vi "Project_Final_2016.vi"() -> ()   [LabVIEW 2015]
uses:
  <vilib>/DAQmx/read.llb/DAQmx Read (Digital Bool 1Line 1Point).vi
  <vilib>/DAQmx/write.llb/DAQmx Write (Digital Bool 1Line 1Point).vi
  <vilib>/DAQmx/create/channels.llb/DAQmx Create Channel (DI-Digital Input).vi
  <vilib>/DAQmx/create/channels.llb/DAQmx Create Channel (DO-Digital Output).vi
  <vilib>/DAQmx/miscellaneous.llb/DAQmx Fill In Error Info.vi
  <vilib>/Utility/file.llb/Read Delimited Spreadsheet (DBL).vi
  <vilib>/Utility/file.llb/Write Delimited Spreadsheet (DBL).vi
panel:
  out "Reject area solenoid return":bool=TRUE
  out "Rejecting \nBelt Solenoid":bool
  out "Rotary Solenoid":bool
  out "Solenoid Return Sensor":bool=TRUE
  out "Sorting \nChain Solenoid":bool
  in  "BELT":bool
  in  "CHAIN":bool
  in  "PAUSE":bool
  in  "On/Off":bool
  out "cluster 2":T1
  out "ARRAY 2":dbl[](array[numeric])
  in  "Destination 2":path=path "C:/Users/dnt4/Downloads/data2.txt"
  out "ARRAY":dbl[](array[numeric])
  out "output cluster 2":T2
  out "output cluster":T3
  out "cluster":T4
  out "sensing area peg detect fake":bool
  in  "stop 4":bool
  in  "Assist sensing loop1 3":bool
  out "reject wait":dbl
  out "reject assistant":dbl
  in  "Assist sensing loop1 2":bool
  out "protection":dbl
  in  "stop 3":bool
  out "Assembly detect fake":bool
  out "Emergency Stop ACTIVATED":bool
  in  "Store Values":bool
  in  "Restore Values":bool
  out "Fake Emergency stop":bool
  out "% Efficiency":dbl(slide) scale=0.0..1.0 scale format="%.2f"
  in  "Clear":bool
  in  "stop 2":bool
  in  "Power Failure":bool
  out "array 2":dbl[](array[numeric])
  in  "Destination 1":path=path "C:/Users/dnt4/Downloads/data1.txt"
  out "array":dbl[](array[numeric])
  out "Stopped":bool=TRUE
  in  "stop AddOn Reject 1":bool
  out "Assembly Assist":dbl
  in  "Assist sensing loop1":bool
  in  "stop sensing station":bool
  out "Assembly Detect":bool
  out "# of Assembly Made":dbl(slide) scale=0.0..20.0
  out "# of Rings Rejected":dbl(slide) scale=0.0..20.0
  out "# of Peg Rejected":dbl(slide) scale=0.0..20.0
  out "# of Ring in the chute":dbl(slide) scale=0.0..5.0
  in  "stop reject area":bool
  out "Reject Area Detected":bool
  out "Sensing Area\n Peg Detected":bool
  out "Sensing Area \nRing Detected":bool
  in  "stop sensing area":bool
  out "Hopper is FULL":bool=TRUE
  in  "stop assembly chute":bool
  out "Sorting Area \nPeg detect":bool
  out "Sorting Area \nPart Detect":bool
  out "Running":bool
  in  "stop":bool
  # "Industrial Control  Trainer (ICT) USER CONTROL PANEL"
  # "Solenoid Activity"
  # "DATA STORAGE LOCATION"
  # "CHAIN/BELT CONTROL"
  # "Main Control"
  # "Sensor Activities"
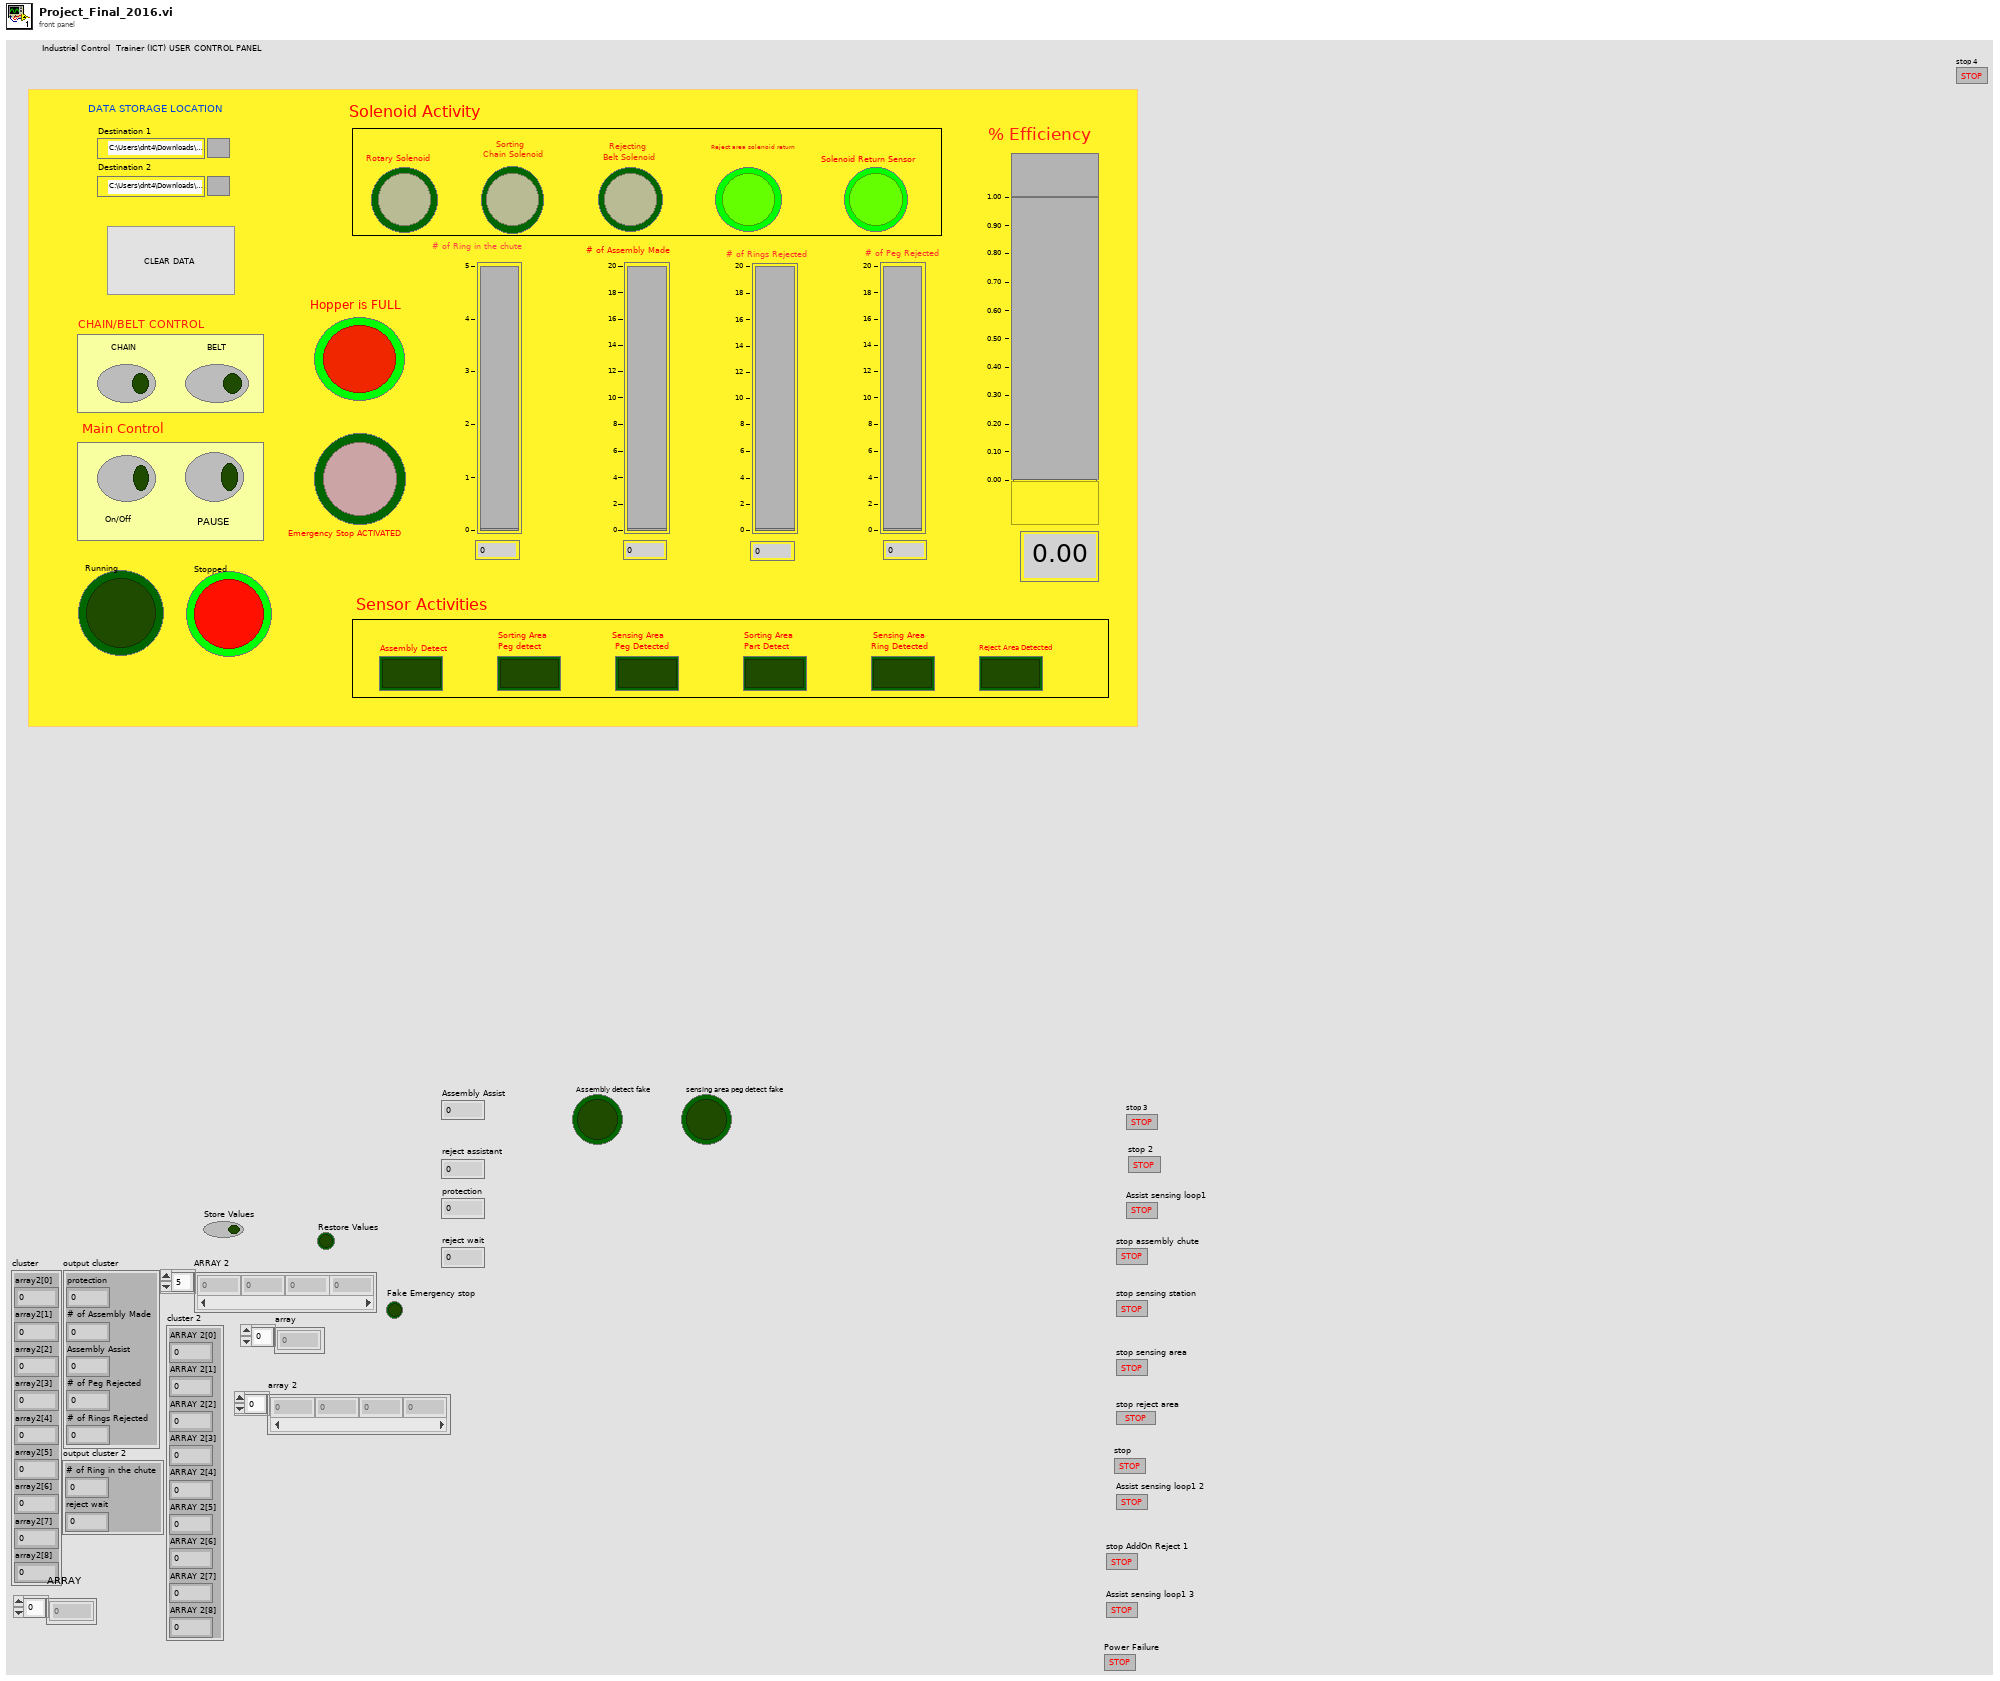
[diagram p1: front panel]
types:
  T1 = cluster{"ARRAY 2[0]":dbl, "ARRAY 2[1]":dbl, "ARRAY 2[2]":dbl, "ARRAY 2[3]":dbl, "ARRAY 2[4]":dbl, "ARRAY 2[5]":dbl, "ARRAY 2[6]":dbl, "ARRAY 2[7]":dbl, "ARRAY 2[8]":dbl}
  T2 = cluster{"# of Ring in the chute":dbl, "reject wait":dbl}
  T3 = cluster{"protection":dbl, "# of Assembly Made":dbl, "Assembly Assist":dbl, "# of Peg Rejected":dbl, "# of Rings Rejected":dbl}
  T4 = cluster{"array2[0]":dbl, "array2[1]":dbl, "array2[2]":dbl, "array2[3]":dbl, "array2[4]":dbl, "array2[5]":dbl, "array2[6]":dbl, "array2[7]":dbl, "array2[8]":dbl}
  T5 = cluster{"array 2[0]":dbl, "array 2[1]":dbl, "array 2[2]":dbl, "array 2[3]":dbl, "array 2[4]":dbl, "array 2[5]":dbl, "array 2[6]":dbl, "array 2[7]":dbl, "array 2[8]":dbl}
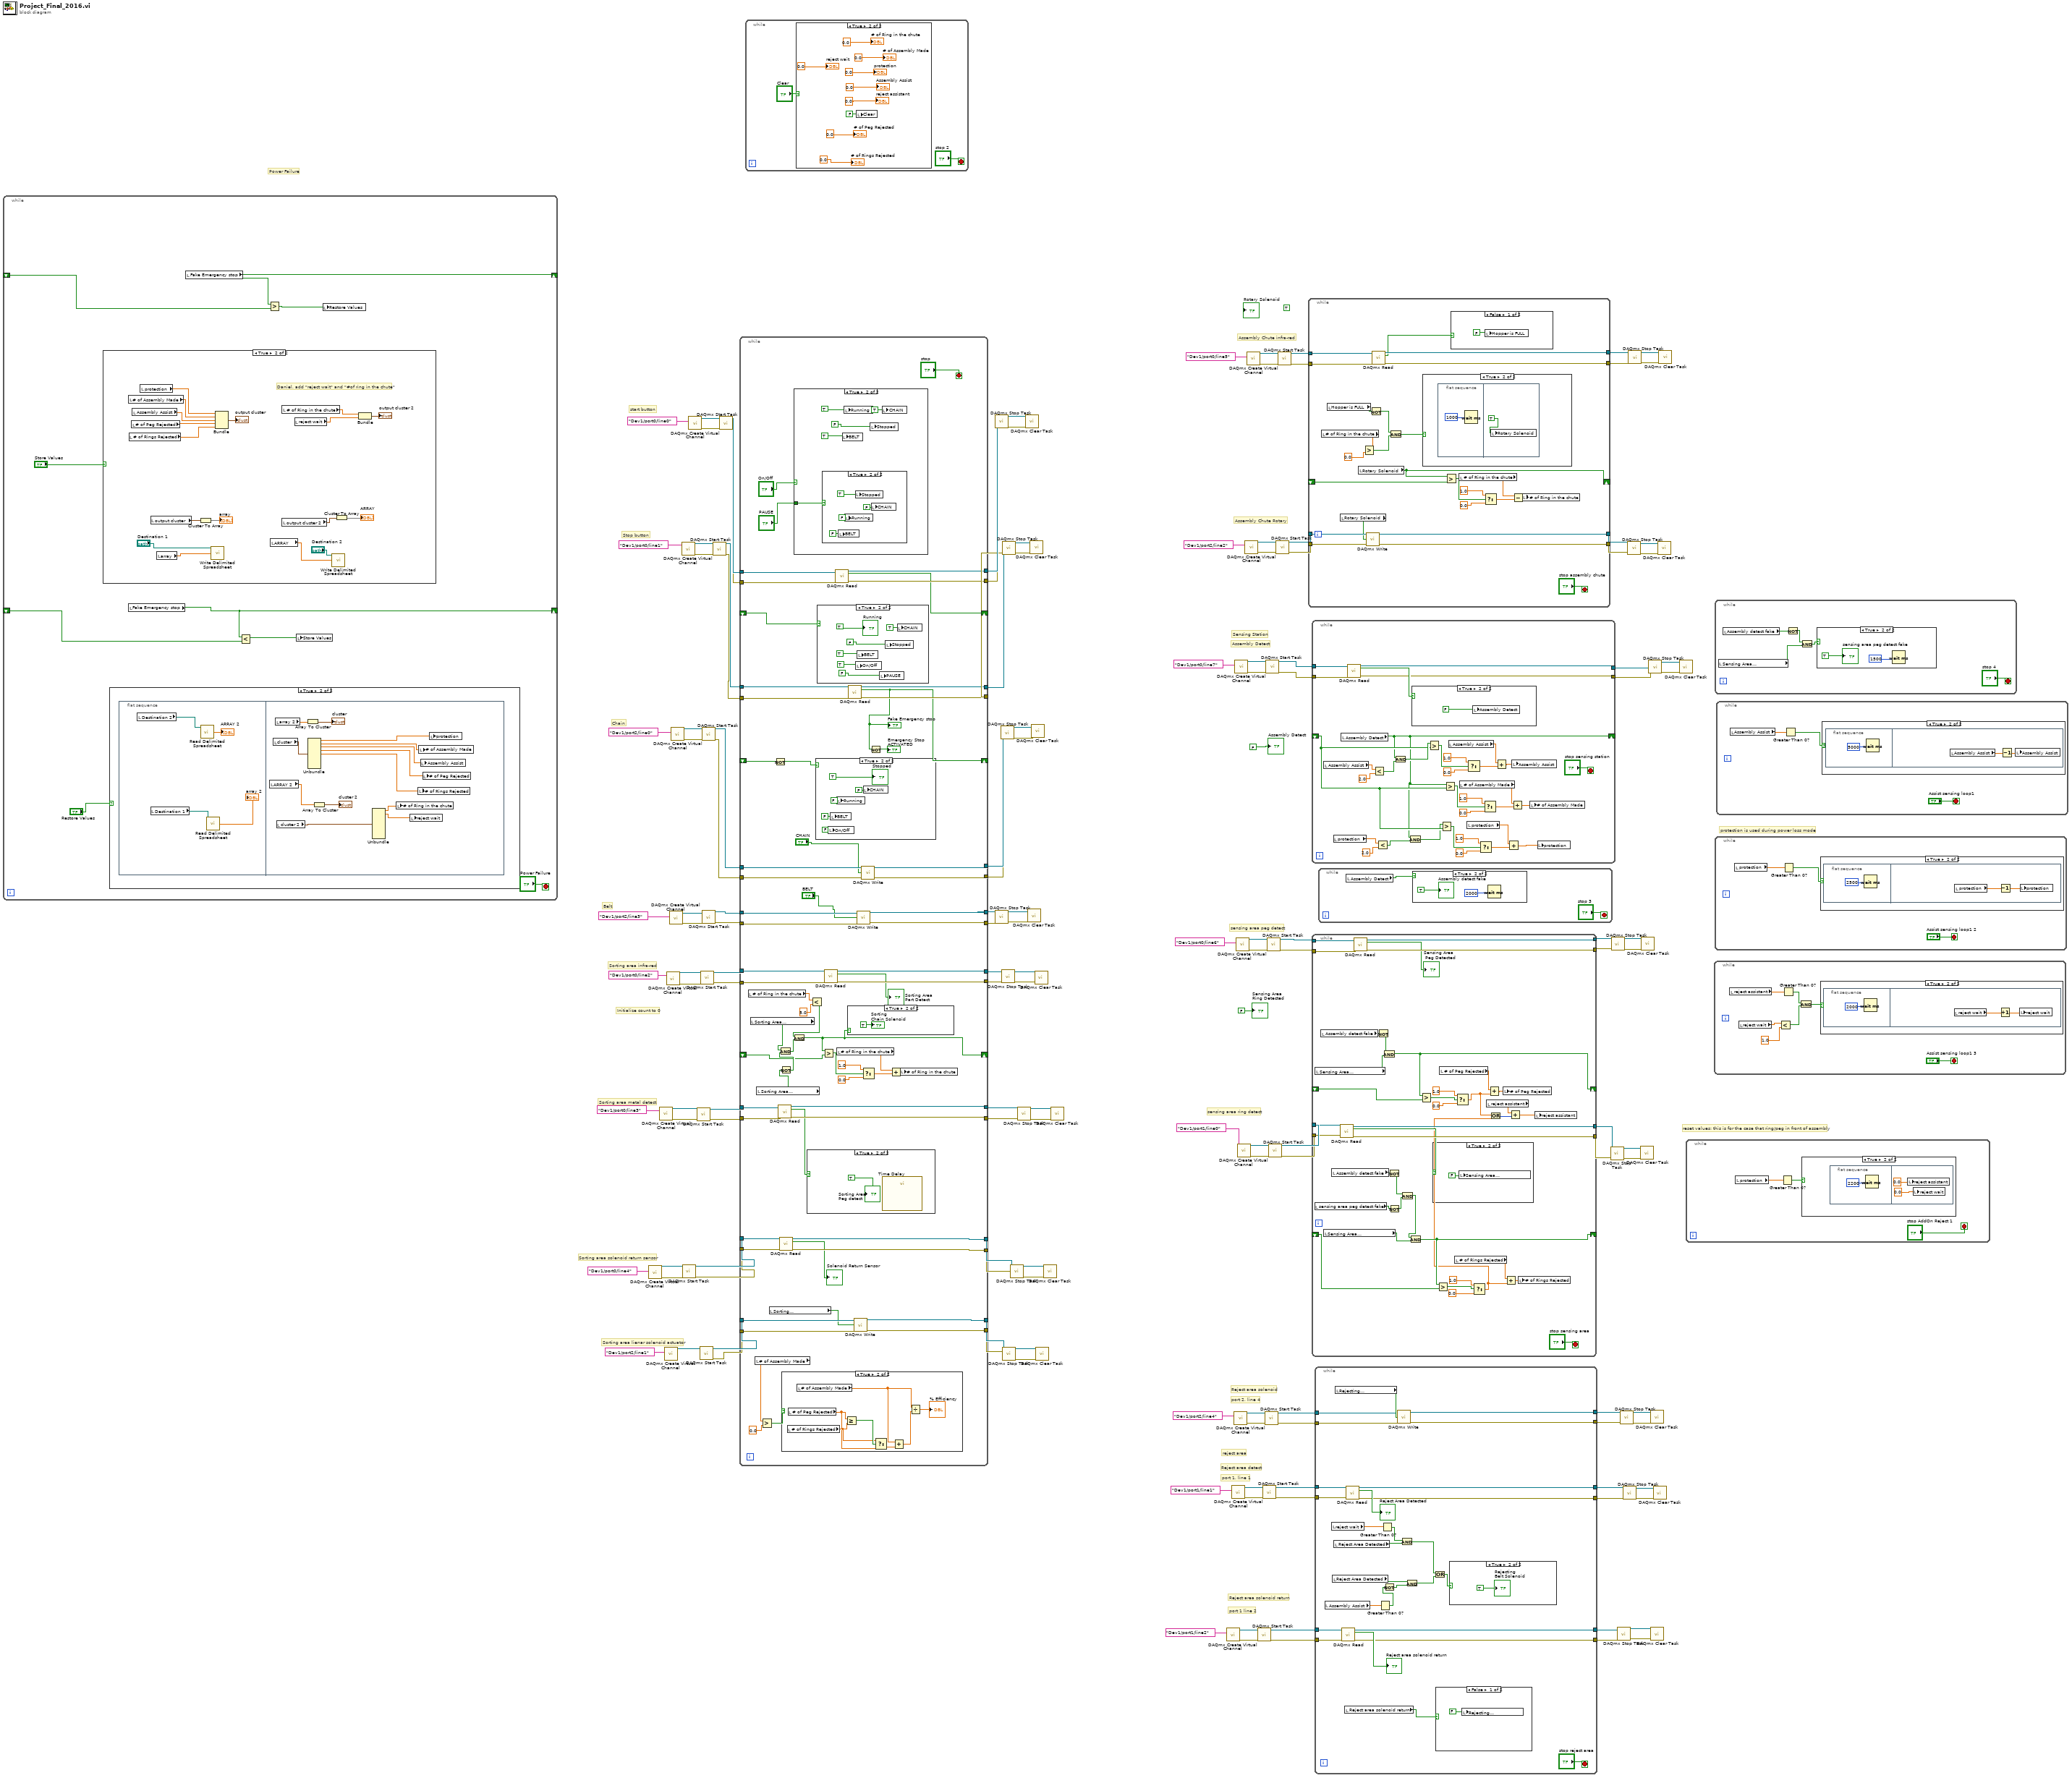
[diagram p0: block diagram]
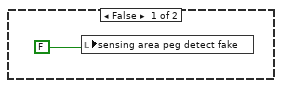
[diagram p4: hidden frame]
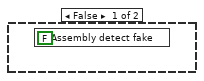
[diagram p7: hidden frame]
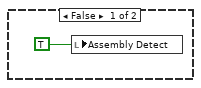
[diagram p11: hidden frame]
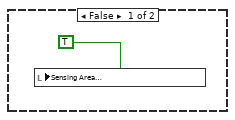
[diagram p14: hidden frame]
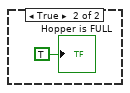
[diagram p15: hidden frame]
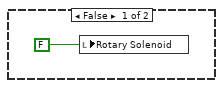
[diagram p16: hidden frame]
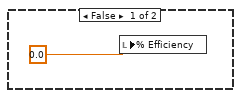
[diagram p17: hidden frame]
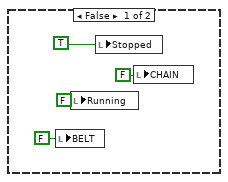
[diagram p18: hidden frame]
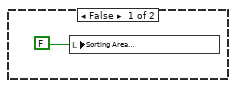
[diagram p20: hidden frame]
diagram:
  (unwired) TRUE
  # "protection is used during power loss mode"
  # "Power Failure"
  # "reset values: this is for the case that ring/peg in front of assembly"
  # "port 1 line 2"
  # "Reject area solenoid return"
  # "Assembly Detect"
  # "Sensing Station"
  # "port 1, line 1"
  # "Reject area detect"
  # "reject area"
  # "port 2, line 4"
  # "Reject area solenoid"
  # "sensing area ring detect"
  # "sensing area peg detect"
  # "Assembly Chute Rotary"
  # "Assembly Chute infra-red"
  # "Sorting area lienar solenoid actuator"
  # "Sorting area solenoid return sensor"
  # "Initialize count to 0"
  # "Sorting area metal detect"
  # "Sorting area infra-red"
  # "Belt"
  # "Chain"
  # "Stop button"
  # "start button"
  n1 = while {
    shift-right: [w152] -> _
    shift-left: _ -> [w153]
    shift-right: [w150] -> _
    shift-left: _ -> [w149]
    stop <- "Power Failure" stop-if-true
    n2 = case shown="True" "Store Values" {
      frame False {
      }
      frame True {
        # "Daniel, add \"reject wait\" and \"#of ring in the chute\""
        n3 = local read "# of Assembly Made"() -> (w170:dbl)
        n4 = local read "# of Rings Rejected"() -> (w167:dbl)
        n5 = local read "# of Peg Rejected"() -> (w168:dbl)
        n6 = local read "Assembly Assist"() -> (w169:dbl)
        n7 = local read "protection"() -> (w171:dbl)
        n8 = local read "output cluster"() -> (w160:T3)
        n9 = local read "array"() -> (w165:dbl[])
        n10 = Cluster To Array(cluster=w160) -> (array=→"array":dbl[])
        n11 = call-poly <vilib>:"Write Delimited Spreadsheet.vi"("file path (dialog if empty)"="Destination 1", "1D data"=w165) -> ()  [unwired: 12 in, 2 out]
        n12 = Bundle("protection"=w171, "# of Assembly Made"=w170, "Assembly Assist"=w169, "# of Peg Rejected"=w168, "# of Rings Rejected"=w167) -> (→"output cluster":T3)  [unwired: 1 in]
        n13 = local read "ARRAY"() -> (w156:dbl[])
        n14 = local read "# of Ring in the chute"() -> (w163:dbl)
        n15 = local read "output cluster 2"() -> (w158:T2)
        n16 = local read "reject wait"() -> (w162:dbl)
        n17 = call-poly <vilib>:"Write Delimited Spreadsheet.vi"("file path (dialog if empty)"="Destination 2", "1D data"=w156) -> ()  [unwired: 12 in, 2 out]
        n18 = Cluster To Array(cluster=w158) -> (array=→"ARRAY":dbl[])
        n19 = Bundle("# of Ring in the chute"=w163, "reject wait"=w162) -> (→"output cluster 2":T2)  [unwired: 1 in]
      }
    }
    n20 = case shown="True" "Restore Values" {
      frame False {
      }
      frame True {
        n21 = flat-sequence {
          frame #0 {
            n22 = local read "Destination 2"() -> (w172:path)
            n23 = local read "Destination 1"() -> (w174:path)
            n24 = call-poly <vilib>:"Read Delimited Spreadsheet.vi"("file path (dialog if empty)"=w172) -> ("first row"=→"ARRAY 2":dbl[])  [unwired: 9 in, 5 out]
            n25 = call-poly <vilib>:"Read Delimited Spreadsheet.vi"("file path (dialog if empty)"=w174) -> ("first row"=→"array 2":dbl[])  [unwired: 9 in, 5 out]
          }
          frame #1 {
            n26 = local read "ARRAY 2"() -> (w180:dbl[])
            n27 = local read "cluster"() -> (w187:T4)
            n28 = local read "array 2"() -> (w188:dbl[])
            n29 = local read "cluster 2"() -> (w178:T1)
            n30 = Array To Cluster(array=w188) -> (cluster=→"cluster":T5)
            n31 = Unbundle(w187) -> ("array2[0]"=w186:dbl, "array2[1]"=w183:dbl, "array2[2]"=w182:dbl, "array2[3]"=w185:dbl, "array2[4]"=w184:dbl)  [unwired: 4 out]
            n32 = Array To Cluster(array=w180) -> (cluster=→"cluster 2":T1)
            n33 = Unbundle(w178) -> ("ARRAY 2[0]"=w177:dbl, "ARRAY 2[1]"=w176:dbl)  [unwired: 7 out]
            n34 = local write "# of Ring in the chute"(w177) -> ()
            n35 = local write "reject wait"(w176) -> ()
            n36 = local write "# of Rings Rejected"(w184) -> ()
            n37 = local write "# of Assembly Made"(w183) -> ()
            n38 = local write "Assembly Assist"(w182) -> ()
            n39 = local write "# of Peg Rejected"(w185) -> ()
            n40 = local write "protection"(w186) -> ()
          }
        }
      }
    }
    n41 = local read "Fake Emergency stop"() -> (w152:bool)
    n42 = local read "Fake Emergency stop"() -> (w150:bool)
    n43 = Less?(x=w152, y=w153) -> (x < y?=w147:bool)
    n44 = Greater?(x=w150, y=w149) -> (0:w148:bool)
    n45 = local write "Store Values"(w147) -> ()
    n46 = local write "Restore Values"(w148) -> ()
  }
  n47 = call-poly <vilib>:"DAQmx Create Virtual Channel.vi"("lines"=tag "Dev1/port0/line4") -> ("task out"=w91:refnum<k21>, "error out"=w90:errorcluster)  [unwired: 13 in]
  n48 = call-poly <vilib>:"DAQmx Create Virtual Channel.vi"("lines"=tag "Dev1/port0/line3") -> ("task out"=w82:refnum<k21>, "error out"=w78:errorcluster)  [unwired: 13 in]
  n49 = call-poly <vilib>:"DAQmx Create Virtual Channel.vi"("lines"=tag "Dev1/port2/line1") -> ("task out"=w99:refnum<k21>)  [unwired: 13 in, 1 out]
  n50 = call-poly <vilib>:"DAQmx Create Virtual Channel.vi"("lines"=tag "Dev1/port0/line2") -> ("task out"=w108:refnum<k21>, "error out"=w101:errorcluster)  [unwired: 13 in]
  n51 = call-poly <vilib>:"DAQmx Create Virtual Channel.vi"("lines"=tag "Dev1/port2/line3") -> ("task out"=w117:refnum<k21>, "error out"=w114:errorcluster)  [unwired: 13 in]
  n52 = call-poly <vilib>:"DAQmx Create Virtual Channel.vi"("lines"=tag "Dev1/port2/line0") -> ("task out"=w126:refnum<k21>, "error out"=w125:errorcluster)  [unwired: 13 in]
  n53 = call-poly <vilib>:"DAQmx Create Virtual Channel.vi"("lines"=tag "Dev1/port0/line1") -> ("task out"=w135:refnum<k21>, "error out"=w134:errorcluster)  [unwired: 13 in]
  n54 = call <vilib>:"DAQmx Start Task.vi"("task/channels in"=w91, "error in"=w90) -> ("task out"=w89:refnum<k21>, "error out"=w84:errorcluster)  [unwired: 12 in]
  n55 = call-poly <vilib>:"DAQmx Create Virtual Channel.vi"("lines"=tag "Dev1/port0/line0") -> ("task out"=w144:refnum<k21>, "error out"=w140:errorcluster)  [unwired: 13 in]
  n56 = call <vilib>:"DAQmx Start Task.vi"("task/channels in"=w82, "error in"=w78) -> ("task out"=w79:refnum<k21>, "error out"=w77:errorcluster)  [unwired: 12 in]
  n57 = call <vilib>:"DAQmx Start Task.vi"("task/channels in"=w99) -> ("task out"=w98:refnum<k21>, "error out"=w95:errorcluster)  [unwired: 13 in]
  n58 = call <vilib>:"DAQmx Start Task.vi"("task/channels in"=w108, "error in"=w101) -> ("task out"=w107:refnum<k21>, "error out"=w104:errorcluster)  [unwired: 12 in]
  n59 = call <vilib>:"DAQmx Start Task.vi"("task/channels in"=w126, "error in"=w125) -> ("task out"=w122:refnum<k21>, "error out"=w120:errorcluster)  [unwired: 12 in]
  n60 = call <vilib>:"DAQmx Start Task.vi"("task/channels in"=w117, "error in"=w114) -> ("task out"=w116:refnum<k21>, "error out"=w113:errorcluster)  [unwired: 12 in]
  n61 = call <vilib>:"DAQmx Start Task.vi"("task/channels in"=w135, "error in"=w134) -> ("task out"=w131:refnum<k21>, "error out"=w130:errorcluster)  [unwired: 12 in]
  n62 = call <vilib>:"DAQmx Start Task.vi"("task/channels in"=w144, "error in"=w140) -> ("task out"=w143:refnum<k21>, "error out"=w139:errorcluster)  [unwired: 12 in]
  n63 = while {
    tunnel: w143 -> [w196]
    tunnel: [w253] -> w142
    tunnel: w139 -> [w252]
    tunnel: [w251] -> w138
    shift-right: [w249] -> _
    shift-left: _ -> [w199]
    tunnel: w131 -> [w248]
    tunnel: w130 -> [w247]
    tunnel: [w246] -> w129
    tunnel: [w245] -> w128
    shift-right: [w189] -> _
    shift-left: _ -> [w244]
    tunnel: w122 -> [w242]
    tunnel: [w241] -> w121
    tunnel: w120 -> [w240]
    tunnel: [w239] -> w119
    tunnel: w116 -> [w238]
    tunnel: [w237] -> w115
    tunnel: w113 -> [w236]
    tunnel: [w235] -> w112
    tunnel: w107 -> [w234]
    tunnel: [w233] -> w106
    tunnel: w104 -> [w232]
    tunnel: [w231] -> w103
    tunnel: w98 -> [w230]
    tunnel: [w229] -> w97
    tunnel: w95 -> [w228]
    tunnel: [w227] -> w94
    tunnel: w89 -> [w225]
    tunnel: [w224] -> w86
    tunnel: [w223] -> w85
    tunnel: w84 -> [w222]
    tunnel: w79 -> [w221]
    tunnel: w77 -> [w220]
    tunnel: [w219] -> w76
    tunnel: [w217] -> w75
    shift-right: [w206] -> _
    shift-left: _ -> [w207]
    stop <- "stop" stop-if-true
    n64 = local read "# of Ring in the chute"() -> (w212:dbl)
    n65 = local read "Sorting Area \nPart Detect"() -> (w208:bool)
    n66 = local read "# of Assembly Made"() -> (w193:dbl)
    n67 = local read "Sorting Area \nPeg detect"() -> (w216:bool)
    n68 = Greater?(x=w193, y=0.0) -> (0:w191:bool)
    n69 = local read "Sorting \nChain Solenoid"() -> (w226:bool)
    n70 = Not(x=w244) -> (.not. x?=w243:bool)
    n71 = call-poly <vilib>:"DAQmx Read.vi"("task/channels in"=w221, "error in"=w220) -> ("task out"=w217:refnum<k21>, "data"=w218:bool, "error out"=w219:errorcluster)  [unwired: 11 in]
    n72 = call-poly <vilib>:"DAQmx Read.vi"("task/channels in"=w225, "error in"=w222) -> ("task out"=w224:refnum<k21>, "data"=→"Solenoid Return Sensor":bool, "error out"=w223:errorcluster)  [unwired: 11 in]
    n73 = Not(x=w216) -> (.not. x?=w215:bool)
    n74 = And(x=w208, y=w215) -> (x .and. y?=w214:bool)
    n75 = case shown="True" w191 {
      frame False {
        n76 = local write "% Efficiency"(0.0) -> ()
      }
      frame True {
        n77 = local read "# of Rings Rejected"() -> (w260:dbl)
        n78 = local read "# of Peg Rejected"() -> (w259:dbl)
        n79 = local read "# of Assembly Made"() -> (w256:dbl)
        n80 = Greater Or Equal?(x=w259, y=w260) -> (x >= y?=w261:bool)
        n81 = Select(t=w260, s=w261, f=w259) -> (s? t:f=w257:dbl)
        n82 = Add(x=w256, y=w257) -> (x+y=w255:dbl)
        n83 = Divide(x=w256, y=w255) -> (x/y=→"% Efficiency":dbl)
      }
    }
    n84 = case shown="True" "On/Off" {
      tunnel: "PAUSE" -> [_ w266]
      frame False {
        n85 = local write "BELT"(FALSE ("belt")) -> ()
        n86 = local write "Running"(FALSE ("Start")) -> ()
        n87 = local write "Stopped"(TRUE ("Stop")) -> ()
        n88 = local write "CHAIN"(FALSE) -> ()
      }
      frame True {
        n89 = case shown="True" w266 {
          frame False {
          }
          frame True {
            n90 = local write "BELT"(FALSE ("belt")) -> ()
            n91 = local write "Running"(FALSE ("Start")) -> ()
            n92 = local write "Stopped"(TRUE ("Stop")) -> ()
            n93 = local write "CHAIN"(FALSE) -> ()
          }
        }
        n94 = local write "BELT"(TRUE) -> ()
        n95 = local write "Running"(TRUE) -> ()
        n96 = local write "Stopped"(FALSE) -> ()
        n97 = local write "CHAIN"(TRUE) -> ()
      }
    }
    n98 = case shown="True" w218 {
      frame False {
        n99 = local write "Sorting Area \nPeg detect"(FALSE) -> ()
      }
      frame True {
        n100 = call "Time Delay"() -> ()  [unwired: 11 in, 1 out]
        "Sorting Area \nPeg detect" <- TRUE
      }
    }
    n101 = Less?(x=w212, y=5.0) -> (x < y?=w211:bool)
    n102 = And(x=w211, y=w214) -> (x .and. y?=w206:bool)
    n103 = case shown="True" w243 {
      frame False {
      }
      frame True {
        n104 = local write "On/Off"(FALSE ("belt")) -> ()
        n105 = local write "BELT"(FALSE ("belt")) -> ()
        n106 = local write "Running"(FALSE ("Start")) -> ()
        n107 = local write "CHAIN"(FALSE) -> ()
        "Stopped" <- TRUE ("Stop")
      }
    }
    n108 = case shown="True" w199 {
      frame False {
      }
      frame True {
        n109 = local write "On/Off"(TRUE) -> ()
        n110 = local write "BELT"(TRUE) -> ()
        n111 = local write "PAUSE"(FALSE) -> ()
        n112 = local write "Stopped"(FALSE) -> ()
        n113 = local write "CHAIN"(TRUE) -> ()
        "Running" <- TRUE
      }
    }
    n114 = Greater?(x=w206, y=w207) -> (0:w203:bool)
    n115 = call-poly <vilib>:"DAQmx Read.vi"("task/channels in"=w234, "error in"=w232) -> ("task out"=w233:refnum<k21>, "data"=→"Sorting Area \nPart Detect":bool, "error out"=w231:errorcluster)  [unwired: 11 in]
    n116 = call-poly <vilib>:"DAQmx Read.vi"("task/channels in"=w196, "error in"=w252) -> ("task out"=w253:refnum<k21>, "data"=w249:bool, "error out"=w251:errorcluster)  [unwired: 11 in]
    n117 = local read "# of Ring in the chute"() -> (w200:dbl)
    n118 = case shown="True" w206 {
      frame False {
        n119 = local write "Sorting \nChain Solenoid"(FALSE) -> ()
      }
      frame True {
        "Sorting \nChain Solenoid" <- TRUE
      }
    }
    n120 = call-poly <vilib>:"DAQmx Read.vi"("task/channels in"=w248, "error in"=w247) -> ("task out"=w246:refnum<k21>, "data"=w189:bool, "error out"=w245:errorcluster)  [unwired: 11 in]
    "Fake Emergency stop" <- w189
    n121 = call-poly <vilib>:"DAQmx Write.vi"("task/channels in"=w230, "data"=w226, "error in"=w228) -> ("task out"=w229:refnum<k21>, "error out"=w227:errorcluster)  [unwired: 10 in, 1 out]
    n122 = call-poly <vilib>:"DAQmx Write.vi"("task/channels in"=w238, "data"="BELT", "error in"=w236) -> ("task out"=w237:refnum<k21>, "error out"=w235:errorcluster)  [unwired: 10 in, 1 out]
    n123 = call-poly <vilib>:"DAQmx Write.vi"("task/channels in"=w242, "data"="CHAIN", "error in"=w240) -> ("task out"=w241:refnum<k21>, "error out"=w239:errorcluster)  [unwired: 10 in, 1 out]
    n124 = Select(t=1.0, s=w203, f=0.0) -> (s? t:f=w202:dbl)
    n125 = Not(x=w189) -> (.not. x?=→"Emergency Stop ACTIVATED":bool)
    n126 = Add(x=w200, y=w202) -> (x+y=w201:dbl)
    n127 = local write "# of Ring in the chute"(w201) -> ()
  }
  n128 = while {
    stop <- "stop 2" stop-if-true
    n129 = case shown="True" "Clear" {
      frame False {
      }
      frame True {
        n130 = local write "Clear"(FALSE ("Clear")) -> ()
        "# of Ring in the chute" <- 0.0
        "# of Peg Rejected" <- 0.0
        "# of Rings Rejected" <- 0.0
        "# of Assembly Made" <- 0.0
        "Assembly Assist" <- 0.0
        "protection" <- 0.0
        "reject assistant" <- 0.0
        "reject wait" <- 0.0
      }
    }
  }
  n131 = call <vilib>:"DAQmx Stop Task.vi"("task/channels in"=w115, "error in"=w112) -> ("task out"=w110:refnum<k21>, "error out"=w111:errorcluster)  [unwired: 12 in]
  n132 = call <vilib>:"DAQmx Stop Task.vi"("task/channels in"=w142, "error in"=w138) -> ("task out"=w141:refnum<k21>, "error out"=w137:errorcluster)  [unwired: 12 in]
  n133 = call <vilib>:"DAQmx Stop Task.vi"("task/channels in"=w121, "error in"=w119) -> ("task out"=w124:refnum<k21>, "error out"=w123:errorcluster)  [unwired: 12 in]
  n134 = call <vilib>:"DAQmx Stop Task.vi"("task/channels in"=w106, "error in"=w103) -> ("task out"=w105:refnum<k21>, "error out"=w102:errorcluster)  [unwired: 12 in]
  n135 = call <vilib>:"DAQmx Stop Task.vi"("task/channels in"=w129, "error in"=w128) -> ("task out"=w133:refnum<k21>, "error out"=w132:errorcluster)  [unwired: 12 in]
  n136 = call <vilib>:"DAQmx Stop Task.vi"("task/channels in"=w97, "error in"=w94) -> ("task out"=w96:refnum<k21>, "error out"=w93:errorcluster)  [unwired: 12 in]
  n137 = call <vilib>:"DAQmx Stop Task.vi"("task/channels in"=w86, "error in"=w85) -> ("task out"=w88:refnum<k21>, "error out"=w87:errorcluster)  [unwired: 12 in]
  n138 = call <vilib>:"DAQmx Stop Task.vi"("task/channels in"=w75, "error in"=w76) -> ("task out"=w81:refnum<k21>, "error out"=w80:errorcluster)  [unwired: 12 in]
  n139 = call <vilib>:"DAQmx Clear Task.vi"("task in"=w141, "error in"=w137) -> ()  [unwired: 13 in, 1 out]
  n140 = call <vilib>:"DAQmx Clear Task.vi"("task in"=w110, "error in"=w111) -> ()  [unwired: 13 in, 1 out]
  n141 = call <vilib>:"DAQmx Clear Task.vi"("task in"=w133, "error in"=w132) -> ()  [unwired: 13 in, 1 out]
  n142 = call <vilib>:"DAQmx Clear Task.vi"("task in"=w124, "error in"=w123) -> ()  [unwired: 13 in, 1 out]
  n143 = call <vilib>:"DAQmx Clear Task.vi"("task in"=w105, "error in"=w102) -> ()  [unwired: 13 in, 1 out]
  n144 = call <vilib>:"DAQmx Clear Task.vi"("task in"=w96, "error in"=w93) -> ()  [unwired: 13 in, 1 out]
  n145 = call <vilib>:"DAQmx Clear Task.vi"("task in"=w88, "error in"=w87) -> ()  [unwired: 13 in, 1 out]
  n146 = call <vilib>:"DAQmx Clear Task.vi"("task in"=w81, "error in"=w80) -> ()  [unwired: 13 in, 1 out]
  n147 = call-poly <vilib>:"DAQmx Create Virtual Channel.vi"("lines"=tag "Dev1/port1/line2") -> ("task out"=w10:refnum<k21>, "error out"=w9:errorcluster)  [unwired: 13 in]
  n148 = call-poly <vilib>:"DAQmx Create Virtual Channel.vi"("lines"=tag "Dev1/port1/line1") -> ("task out"=w26:refnum<k21>, "error out"=w27:errorcluster)  [unwired: 13 in]
  n149 = call-poly <vilib>:"DAQmx Create Virtual Channel.vi"("lines"=tag "Dev1/port2/line4") -> ("task out"=w35:refnum<k21>, "error out"=w34:errorcluster)  [unwired: 13 in]
  n150 = call-poly <vilib>:"DAQmx Create Virtual Channel.vi"("lines"=tag "Dev1/port0/line7") -> ("task out"=w17:refnum<k21>, "error out"=w18:errorcluster)  [unwired: 13 in]
  n151 = call-poly <vilib>:"DAQmx Create Virtual Channel.vi"("lines"=tag "Dev1/port0/line6") -> ("task out"=w49:refnum<k21>, "error out"=w50:errorcluster)  [unwired: 13 in]
  n152 = call-poly <vilib>:"DAQmx Create Virtual Channel.vi"("lines"=tag "Dev1/port1/line0") -> ("task out"=w42:refnum<k21>, "error out"=w41:errorcluster)  [unwired: 13 in]
  n153 = call-poly <vilib>:"DAQmx Create Virtual Channel.vi"("lines"=tag "Dev1/port2/line2") -> ("task out"=w68:refnum<k21>, "error out"=w67:errorcluster)  [unwired: 13 in]
  n154 = call-poly <vilib>:"DAQmx Create Virtual Channel.vi"("lines"=tag "Dev1/port0/line5") -> ("task out"=w73:refnum<k21>, "error out"=w74:errorcluster)  [unwired: 13 in]
  n155 = call <vilib>:"DAQmx Start Task.vi"("task/channels in"=w10, "error in"=w9) -> ("task out"=w8:refnum<k21>, "error out"=w7:errorcluster)  [unwired: 12 in]
  n156 = call <vilib>:"DAQmx Start Task.vi"("task/channels in"=w26, "error in"=w27) -> ("task out"=w24:refnum<k21>, "error out"=w23:errorcluster)  [unwired: 12 in]
  n157 = call <vilib>:"DAQmx Start Task.vi"("task/channels in"=w35, "error in"=w34) -> ("task out"=w33:refnum<k21>, "error out"=w32:errorcluster)  [unwired: 12 in]
  n158 = call <vilib>:"DAQmx Start Task.vi"("task/channels in"=w17, "error in"=w18) -> ("task out"=w15:refnum<k21>, "error out"=w14:errorcluster)  [unwired: 12 in]
  n159 = call <vilib>:"DAQmx Start Task.vi"("task/channels in"=w49, "error in"=w50) -> ("task out"=w47:refnum<k21>, "error out"=w46:errorcluster)  [unwired: 12 in]
  n160 = call <vilib>:"DAQmx Start Task.vi"("task/channels in"=w42, "error in"=w41) -> ("task out"=w40:refnum<k21>, "error out"=w39:errorcluster)  [unwired: 12 in]
  n161 = call <vilib>:"DAQmx Start Task.vi"("task/channels in"=w68, "error in"=w67) -> ("task out"=w62:refnum<k21>, "error out"=w61:errorcluster)  [unwired: 12 in]
  n162 = call <vilib>:"DAQmx Start Task.vi"("task/channels in"=w73, "error in"=w74) -> ("task out"=w71:refnum<k21>, "error out"=w70:errorcluster)  [unwired: 12 in]
  n163 = while {
    tunnel: w71 -> [w321]
    tunnel: w70 -> [w320]
    tunnel: [w318] -> w64
    tunnel: [w317] -> w63
    tunnel: w62 -> [w316]
    tunnel: w61 -> [w315]
    tunnel: [w313] -> w58
    tunnel: [w312] -> w57
    shift-right: [w302] -> _
    shift-left: _ -> [w303]
    stop <- "stop assembly chute" stop-if-true
    n164 = local read "# of Ring in the chute"() -> (w325:dbl)
    n165 = local read "Hopper is FULL"() -> (w310:bool)
    n166 = local read "Rotary Solenoid"() -> (w314:bool)
    n167 = local read "Rotary Solenoid"() -> (w302:bool)
    n168 = Greater?(x=w325, y=0.0) -> (0:w323:bool)
    n169 = call-poly <vilib>:"DAQmx Write.vi"("task/channels in"=w316, "data"=w314, "error in"=w315) -> ("task out"=w313:refnum<k21>, "error out"=w312:errorcluster)  [unwired: 10 in, 1 out]
    n170 = Not(x=w310) -> (.not. x?=w319:bool)
    n171 = call-poly <vilib>:"DAQmx Read.vi"("task/channels in"=w321, "error in"=w320) -> ("task out"=w318:refnum<k21>, "data"=w311:bool, "error out"=w317:errorcluster)  [unwired: 11 in]
    n172 = And(x=w319, y=w323) -> (x .and. y?=w301:bool)
    n173 = case shown="True" w301 {
      frame False {
        n174 = local write "Rotary Solenoid"(FALSE) -> ()
      }
      frame True {
        n175 = flat-sequence {
          frame #0 {
            n176 = Wait (ms)(milliseconds to wait=u32 1000) -> ()  [unwired: 1 out]
          }
          frame #1 {
            n177 = local write "Rotary Solenoid"(TRUE) -> ()
          }
        }
      }
    }
    n178 = Greater?(x=w302, y=w303) -> (0:w307:bool)
    n179 = case shown="False" w311 {
      frame False {
        n180 = local write "Hopper is FULL"(FALSE) -> ()
      }
      frame True {
        "Hopper is FULL" <- TRUE
      }
    }
    n181 = local read "# of Ring in the chute"() -> (w304:dbl)
    n182 = Select(t=1.0, s=w307, f=0.0) -> (s? t:f=w306:dbl)
    n183 = Subtract(x=w304, y=w306) -> (x-y=w305:dbl)
    n184 = local write "# of Ring in the chute"(w305) -> ()
  }
  n185 = while {
    tunnel: w15 -> [w363]
    tunnel: w14 -> [w362]
    tunnel: [w360] -> w13
    tunnel: [w359] -> w12
    shift-right: [w332] -> _
    shift-left: _ -> [w336]
    stop <- "stop sensing station" stop-if-true
    n186 = local read "Assembly Assist"() -> (w352:dbl)
    n187 = local read "protection"() -> (w334:dbl)
    n188 = local read "Assembly Detect"() -> (w332:bool)
    n189 = call-poly <vilib>:"DAQmx Read.vi"("task/channels in"=w363, "error in"=w362) -> ("task out"=w360:refnum<k21>, "data"=w361:bool, "error out"=w359:errorcluster)  [unwired: 11 in]
    n190 = Less?(x=w352, y=2.0) -> (x < y?=w350:bool)
    n191 = Less?(x=w334, y=2.0) -> (x < y?=w333:bool)
    n192 = And(x=w332, y=w350) -> (x .and. y?=w349:bool)
    n193 = And(x=w332, y=w333) -> (x .and. y?=w331:bool)
    n194 = case shown="True" w361 {
      frame False {
        n195 = local write "Assembly Detect"(TRUE) -> ()
      }
      frame True {
        n196 = local write "Assembly Detect"(FALSE) -> ()
      }
    }
    n197 = Greater?(x=w349, y=w336) -> (0:w356:bool)
    n198 = Greater?(x=w331, y=w336) -> (0:w340:bool)
    n199 = Greater?(x=w332, y=w336) -> (0:w345:bool)
    n200 = local read "Assembly Assist"() -> (w353:dbl)
    n201 = local read "# of Assembly Made"() -> (w348:dbl)
    n202 = local read "protection"() -> (w337:dbl)
    n203 = Select(t=1.0, s=w356, f=0.0) -> (s? t:f=w357:dbl)
    n204 = Select(t=1.0, s=w340, f=0.0) -> (s? t:f=w341:dbl)
    n205 = Select(t=1.0, s=w345, f=0.0) -> (s? t:f=w344:dbl)
    n206 = Add(x=w353, y=w357) -> (x+y=w358:dbl)
    n207 = Add(x=w337, y=w341) -> (x+y=w342:dbl)
    n208 = Add(x=w348, y=w344) -> (x+y=w343:dbl)
    n209 = local write "Assembly Assist"(w358) -> ()
    n210 = local write "# of Assembly Made"(w343) -> ()
    n211 = local write "protection"(w342) -> ()
  }
  n212 = while {
    tunnel: w47 -> [w396]
    tunnel: w46 -> [w395]
    tunnel: [w394] -> w45
    tunnel: [w393] -> w44
    tunnel: w40 -> [w392]
    tunnel: w39 -> [w391]
    tunnel: [w390] -> w38
    tunnel: [w389] -> w37
    shift-right: [w387] -> _
    shift-left: _ -> [w386]
    shift-right: [w374] -> _
    shift-left: _ -> [w375]
    stop <- "stop sensing area" stop-if-true
    n213 = local read "sensing area peg detect fake"() -> (w401:bool)
    n214 = local read "Sensing Area\n Peg Detected"() -> (w403:bool)
    n215 = local read "Assembly detect fake"() -> (w405:bool)
    n216 = local read "Sensing Area \nRing Detected"() -> (w398:bool)
    n217 = local read "Assembly detect fake"() -> (w402:bool)
    n218 = call-poly <vilib>:"DAQmx Read.vi"("task/channels in"=w392, "error in"=w391) -> ("task out"=w390:refnum<k21>, "data"=w388:bool, "error out"=w389:errorcluster)  [unwired: 11 in]
    n219 = call-poly <vilib>:"DAQmx Read.vi"("task/channels in"=w396, "error in"=w395) -> ("task out"=w394:refnum<k21>, "data"=→"Sensing Area\n Peg Detected":bool, "error out"=w393:errorcluster)  [unwired: 11 in]
    n220 = Not(x=w405) -> (.not. x?=w404:bool)
    n221 = And(x=w404, y=w403) -> (x .and. y?=w374:bool)
    n222 = Not(x=w402) -> (.not. x?=w373:bool)
    n223 = Not(x=w401) -> (.not. x?=w400:bool)
    n224 = And(x=w373, y=w400) -> (x .and. y?=w399:bool)
    n225 = And(x=w399, y=w398) -> (x .and. y?=w387:bool)
    n226 = Greater?(x=w374, y=w375) -> (0:w378:bool)
    n227 = case shown="True" w388 {
      frame False {
        n228 = local write "Sensing Area \nRing Detected"(TRUE) -> ()
      }
      frame True {
        n229 = local write "Sensing Area \nRing Detected"(FALSE) -> ()
      }
    }
    n230 = Greater?(x=w387, y=w386) -> (0:w383:bool)
    n231 = local read "# of Peg Rejected"() -> (w379:dbl)
    n232 = local read "# of Rings Rejected"() -> (w382:dbl)
    n233 = Select(t=1.0, s=w378, f=0.0) -> (s? t:f=w369:dbl)
    n234 = Select(t=1.0, s=w383, f=0.0) -> (s? t:f=w368:dbl)
    n235 = local read "reject assistant"() -> (w372:dbl)
    n236 = Add(x=w379, y=w369) -> (x+y=w380:dbl)
    n237 = Or(x=w369, y=w368) -> (x .or. y?=w370:i32)
    n238 = local write "# of Peg Rejected"(w380) -> ()
    n239 = Add(x=w382, y=w368) -> (x+y=w381:dbl)
    n240 = Add(x=w372, y=w370) -> (x+y=w371:dbl)
    n241 = local write "# of Rings Rejected"(w381) -> ()
    n242 = local write "reject assistant"(w371) -> ()
  }
  n243 = while {
    tunnel: w33 -> [w433]
    tunnel: w32 -> [w432]
    tunnel: [w431] -> w29
    tunnel: [w430] -> w28
    tunnel: w24 -> [w428]
    tunnel: w23 -> [w427]
    tunnel: [w426] -> w20
    tunnel: [w425] -> w19
    tunnel: w8 -> [w421]
    tunnel: w7 -> [w420]
    tunnel: [w418] -> w6
    tunnel: [w417] -> w4
    stop <- "stop reject area" stop-if-true
    n244 = local read "Assembly Assist"() -> (w416:dbl)
    n245 = local read "reject wait"() -> (w412:dbl)
    n246 = local read "Reject Area Detected"() -> (w422:bool)
    n247 = local read "Reject Area Detected"() -> (w413:bool)
    n248 = local read "Rejecting \nBelt Solenoid"() -> (w434:bool)
    n249 = call-poly <vilib>:"DAQmx Read.vi"("task/channels in"=w421, "error in"=w420) -> ("task out"=w418:refnum<k21>, "data"=→"Reject area solenoid return":bool, "error out"=w417:errorcluster)  [unwired: 11 in]
    n250 = local read "Reject area solenoid return"() -> (w414:bool)
    n251 = call-poly <vilib>:"DAQmx Read.vi"("task/channels in"=w428, "error in"=w427) -> ("task out"=w426:refnum<k21>, "data"=→"Reject Area Detected":bool, "error out"=w425:errorcluster)  [unwired: 11 in]
    n252 = Greater Than 0?(x=w416) -> (x > 0?=w415:bool)
    n253 = Greater Than 0?(x=w412) -> (x > 0?=w408:bool)
    n254 = Not(x=w415) -> (.not. x?=w423:bool)
    n255 = call-poly <vilib>:"DAQmx Write.vi"("task/channels in"=w433, "data"=w434, "error in"=w432) -> ("task out"=w431:refnum<k21>, "error out"=w430:errorcluster)  [unwired: 10 in, 1 out]
    n256 = And(x=w408, y=w413) -> (x .and. y?=w410:bool)
    n257 = And(x=w422, y=w423) -> (x .and. y?=w411:bool)
    n258 = Or(x=w410, y=w411) -> (x .or. y?=w409:bool)
    n259 = case shown="False" w414 {
      frame False {
        n260 = local write "Rejecting \nBelt Solenoid"(FALSE) -> ()
      }
      frame True {
      }
    }
    n261 = case shown="True" w409 {
      frame False {
      }
      frame True {
        "Rejecting \nBelt Solenoid" <- TRUE
      }
    }
  }
  n262 = while {
    stop <- "stop 3" stop-if-true
    n263 = local read "Assembly Detect"() -> (w438:bool)
    n264 = case shown="True" w438 {
      frame False {
        n265 = local write "Assembly detect fake"(FALSE) -> ()
      }
      frame True {
        n266 = Wait (ms)(milliseconds to wait=2000) -> ()  [unwired: 1 out]
        "Assembly detect fake" <- TRUE
      }
    }
  }
  n267 = call <vilib>:"DAQmx Stop Task.vi"("task/channels in"=w38, "error in"=w37) -> ("task out"=w51:refnum<k21>, "error out"=w52:errorcluster)  [unwired: 12 in]
  n268 = call <vilib>:"DAQmx Stop Task.vi"("task/channels in"=w45, "error in"=w44) -> ("task out"=w54:refnum<k21>, "error out"=w53:errorcluster)  [unwired: 12 in]
  n269 = call <vilib>:"DAQmx Stop Task.vi"("task/channels in"=w6, "error in"=w4) -> ("task out"=w5:refnum<k21>, "error out"=w3:errorcluster)  [unwired: 12 in]
  n270 = call <vilib>:"DAQmx Stop Task.vi"("task/channels in"=w29, "error in"=w28) -> ("task out"=w31:refnum<k21>, "error out"=w30:errorcluster)  [unwired: 12 in]
  n271 = call <vilib>:"DAQmx Stop Task.vi"("task/channels in"=w20, "error in"=w19) -> ("task out"=w21:refnum<k21>, "error out"=w22:errorcluster)  [unwired: 12 in]
  n272 = call <vilib>:"DAQmx Stop Task.vi"("task/channels in"=w58, "error in"=w57) -> ("task out"=w60:refnum<k21>, "error out"=w59:errorcluster)  [unwired: 12 in]
  n273 = call <vilib>:"DAQmx Stop Task.vi"("task/channels in"=w64, "error in"=w63) -> ("task out"=w65:refnum<k21>, "error out"=w66:errorcluster)  [unwired: 12 in]
  n274 = call <vilib>:"DAQmx Clear Task.vi"("task in"=w51, "error in"=w52) -> ()  [unwired: 13 in, 1 out]
  n275 = call <vilib>:"DAQmx Clear Task.vi"("task in"=w54, "error in"=w53) -> ()  [unwired: 13 in, 1 out]
  n276 = call <vilib>:"DAQmx Stop Task.vi"("task/channels in"=w13, "error in"=w12) -> ("task out"=w55:refnum<k21>, "error out"=w56:errorcluster)  [unwired: 12 in]
  n277 = call <vilib>:"DAQmx Clear Task.vi"("task in"=w31, "error in"=w30) -> ()  [unwired: 13 in, 1 out]
  n278 = call <vilib>:"DAQmx Clear Task.vi"("task in"=w5, "error in"=w3) -> ()  [unwired: 13 in, 1 out]
  n279 = call <vilib>:"DAQmx Clear Task.vi"("task in"=w21, "error in"=w22) -> ()  [unwired: 13 in, 1 out]
  n280 = call <vilib>:"DAQmx Clear Task.vi"("task in"=w60, "error in"=w59) -> ()  [unwired: 13 in, 1 out]
  n281 = call <vilib>:"DAQmx Clear Task.vi"("task in"=w65, "error in"=w66) -> ()  [unwired: 13 in, 1 out]
  n282 = call <vilib>:"DAQmx Clear Task.vi"("task in"=w55, "error in"=w56) -> ()  [unwired: 13 in, 1 out]
  n283 = while {
    stop <- "stop AddOn Reject 1" stop-if-true
    n284 = local read "protection"() -> (w443:dbl)
    n285 = Greater Than 0?(x=w443) -> (x > 0?=w442:bool)
    n286 = case shown="True" w442 {
      frame False {
      }
      frame True {
        n287 = flat-sequence {
          frame #0 {
            n288 = Wait (ms)(milliseconds to wait=2200) -> ()  [unwired: 1 out]
          }
          frame #1 {
            n289 = local write "reject assistant"(0.0) -> ()
            n290 = local write "reject wait"(0.0) -> ()
          }
        }
      }
    }
  }
  n291 = while {
    stop <- "Assist sensing loop1 3" stop-if-true
    n292 = local read "reject assistant"() -> (w453:dbl)
    n293 = local read "reject wait"() -> (w452:dbl)
    n294 = Less?(x=w452, y=1.0) -> (x < y?=w450:bool)
    n295 = Greater Than 0?(x=w453) -> (x > 0?=w449:bool)
    n296 = And(x=w449, y=w450) -> (x .and. y?=w448:bool)
    n297 = case shown="True" w448 {
      frame False {
      }
      frame True {
        n298 = flat-sequence {
          frame #0 {
            n299 = Wait (ms)(milliseconds to wait=2000) -> ()  [unwired: 1 out]
          }
          frame #1 {
            n300 = local read "reject wait"() -> (w456:dbl)
            n301 = Increment(x=w456) -> (x+1=w457:dbl)
            n302 = local write "reject wait"(w457) -> ()
          }
        }
      }
    }
  }
  n303 = while {
    stop <- "stop 4" stop-if-true
    n304 = local read "Sensing Area\n Peg Detected"() -> (w458:bool)
    n305 = local read "Assembly detect fake"() -> (w461:bool)
    n306 = Not(x=w461) -> (.not. x?=w459:bool)
    n307 = And(x=w459, y=w458) -> (x .and. y?=w460:bool)
    n308 = case shown="True" w460 {
      frame False {
        n309 = local write "sensing area peg detect fake"(FALSE) -> ()
      }
      frame True {
        n310 = Wait (ms)(milliseconds to wait=1500) -> ()  [unwired: 1 out]
        "sensing area peg detect fake" <- TRUE
      }
    }
  }
  n311 = while {
    stop <- "Assist sensing loop1 2" stop-if-true
    n312 = local read "protection"() -> (w467:dbl)
    n313 = Greater Than 0?(x=w467) -> (x > 0?=w466:bool)
    n314 = case shown="True" w466 {
      frame False {
      }
      frame True {
        n315 = flat-sequence {
          frame #0 {
            n316 = Wait (ms)(milliseconds to wait=2500) -> ()  [unwired: 1 out]
          }
          frame #1 {
            n317 = local read "protection"() -> (w470:dbl)
            n318 = Decrement(x=w470) -> (x-1=w471:dbl)
            n319 = local write "protection"(w471) -> ()
          }
        }
      }
    }
  }
  n320 = while {
    stop <- "Assist sensing loop1" stop-if-true
    n321 = local read "Assembly Assist"() -> (w473:dbl)
    n322 = Greater Than 0?(x=w473) -> (x > 0?=w472:bool)
    n323 = case shown="True" w472 {
      frame False {
      }
      frame True {
        n324 = flat-sequence {
          frame #0 {
            n325 = Wait (ms)(milliseconds to wait=5000) -> ()  [unwired: 1 out]
          }
          frame #1 {
            n326 = local read "Assembly Assist"() -> (w476:dbl)
            n327 = Decrement(x=w476) -> (x-1=w477:dbl)
            n328 = local write "Assembly Assist"(w477) -> ()
          }
        }
      }
    }
  }
  "Assembly Detect" <- FALSE
  "Sensing Area \nRing Detected" <- FALSE
